vi "FRCts_ClientAPI_Team.vi"(8 "Error In":errorcluster, 9 "Resource":string, 10 "Team":T1, 11 "Action":T4) -> (0 "error out":errorcluster, 3 "XML Out":string)   [LabVIEW 2013, in "FRCts_ClientAPI.lvlib"]
doc: "This VI performs either an HTTP Put, Post, Get, or Delete on the Team resource."
uses:
  FRCts_ClientAPI.lvlib
  FRCts_ClientAPI_Collection.ctl
  <vilib>/httpClient/LabVIEWHTTPClient.lvlib
  <vilib>/httpClient/PUTBuffer.vi
  <vilib>/httpClient/POSTBuffer.vi
  FRCts_ClientAPI_Actions.ctl
  Web Methods/source/VI Source/Web Method Public Interface/FRCts20_WebMethods_ctl_teamIdentifier.ctl
  Web Methods/source/VI Source/FRCts20_WebMethods.lvlib
  Web Methods/source/VI Source/Web Method Public Interface/FRCts20_WebMethods_ctl_singleTeam.ctl
  Backend/source/VI Source/FRCts20_Backend_API/FRCts20_Backend_API_SW.ctl
  Backend/source/VI Source/FRCts20_Backend_API/FRCts20_Backend_API.lvlib
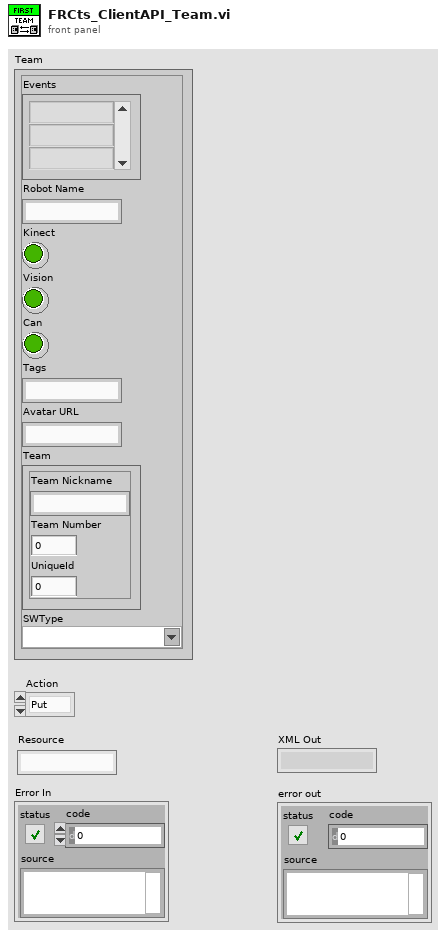
[diagram p1: front panel]
types:
  T1 = typedef "FRCts20_WebMethods.lvlib/FRCts20_WebMethods_ctl_singleTeam.ctl" = cluster{"Events":string[], "Robot Name":string, "Kinect":bool, "Vision":bool, "Can":bool, "Tags":string, "Avatar URL":string, "Team":T2, "SWType":T3}
  T2 = typedef "FRCts20_WebMethods.lvlib/FRCts20_WebMethods_ctl_teamIdentifier.ctl" = cluster{"Team Nickname":string, "Team Number ":u32, "UniqueId":u32}
  T3 = typedef "FRCts20_Backend_API.lvlib/FRCts20_Backend_API_SW.ctl" = string
  T4 = typedef "FRCts_ClientAPI.lvlib/FRCts_ClientAPI_Actions.ctl" = enum16{"Put", "Post", "Get", "Delete"}
  T5 = typedef "FRCts_ClientAPI.lvlib/FRCts_ClientAPI_Collection.ctl" = enum16{"Event", "Events", "Team", "Teams", "Request", "Requests", "Reports"}
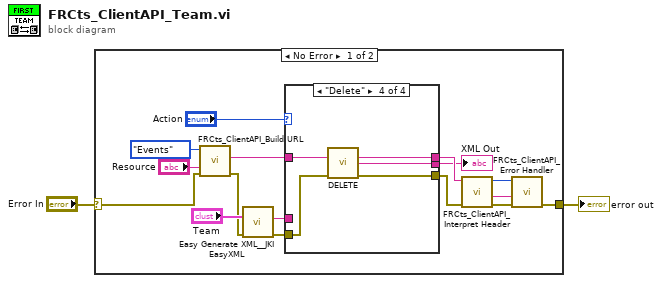
[diagram p0: block diagram]
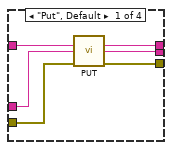
[diagram p2: hidden frame]
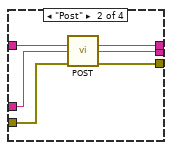
[diagram p3: hidden frame]
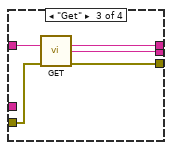
[diagram p4: hidden frame]
diagram:
  n1 = case shown="No Error" "Error In" {
    selector: "Error In" -> [w3 w41]
    tunnel: [w5 w41] -> w2
    frame No Error {
      n2 = call "FRCts_ClientAPI_Build URL.vi"("error in"=w3, "Resource"="Resource", "Collection"=FRCts_ClientAPI_Collection."Events" ("Resource")) -> ("error out"=w4:errorcluster, "URL"=w7:string)  [unwired: 7 in]
      n3 = call <vilib>:"Easy Generate XML__JKI EasyXML.vi"("error in (no error)"=w4, "LabVIEW Data"="Team") -> ("error out"=w10:errorcluster, "XML String"=w9:string)  [unwired: 8 in]
      n4 = case shown="\"Delete\"" "Action" {
        tunnel: w7 -> [w24 w30 w35 w40]
        tunnel: [w23 w28 w34 w39] -> w11
        tunnel: [w22 w29 w33 w38] -> w17
        tunnel: w9 -> [w21 w26 _ _]
        tunnel: w10 -> [w20 w27 w32 w37]
        tunnel: [w19 w25 w31 w36] -> w18
        frame "Put", Default {
          n5 = call-poly <vilib>:"PUT.vi"("url"=w24, "buffer"=w21, "error in (no error)"=w20) -> ("headers"=w19:string, "body"=w23:string, "error out"=w22:errorcluster)  [unwired: 9 in, 1 out]
        }
        frame "Post" {
          n6 = call-poly <vilib>:"POST.vi"("url"=w30, "buffer"=w26, "error in (no error)"=w27) -> ("headers"=w25:string, "body"=w28:string, "error out"=w29:errorcluster)  [unwired: 9 in, 1 out]
        }
        frame "Get" {
          n7 = call <vilib>:"GET.vi"("url"=w35, "error in (no error)"=w32) -> ("headers"=w31:string, "body"=w34:string, "error out"=w33:errorcluster)  [unwired: 10 in, 1 out]
        }
        frame "Delete" {
          n8 = call <vilib>:"DELETE.vi"("url"=w40, "error in (no error)"=w37) -> ("headers"=w36:string, "body"=w39:string, "error out"=w38:errorcluster)  [unwired: 10 in, 1 out]
        }
      }
      "XML Out" <- w11
      n9 = call "FRCts_ClientAPI_Interpret Header.vi"("error in (no error)"=w17, "Header"=w18) -> ("error out"=w15:errorcluster, "HTTP Response"=w16:string, "HTTP Code"=w14:i32)  [unwired: 7 in]
      n10 = call "FRCts_ClientAPI_Error Handler.vi"("error in (no error)"=w15, "HTTP Response"=w16, "HTTP Code"=w14) -> ("error out"=w5:errorcluster)  [unwired: 8 in]
    }
    frame Error {
    }
  }
  "error out" <- w2
